vi "SMO.TimedLoop.TestLauncher.vi"() -> ()   [LabVIEW 2013, in "SMO.TimedLoop.lvclass"]
doc: "JKI State Machine Objects (SMO) 1.0.0.5\nJKI - JKI\nCopyright (c) 2016, JKI"
uses:
  SMO.TimedLoop.lvclass
  Typedefs/Data.ctl
  <vilib>/JKI/JKI SMO/SMO/Typedefs/SMOState --Enum.ctl
  <vilib>/JKI/JKI SMO/SMO/SMO.lvclass
panel:
  out "Value":T1
  in  "Setpoint":dbl(slide) scale=0.0..10.0
  out "error out":errorcluster
  in  "Stop":bool
  # "Timed Loop Test Launcher"
  # "For instructions on how to use the JKI State Machine Objects, examples and video tutorials, visit:\nhttp://jki.net/state-machine-objects/\n\nJKI State Machine Objects™\nhttp://jki.net/state-machine-objects/\nCopyright (C) 2005-2015, JKI <info@jki.net>\nALL RIGHTS RESERVED"
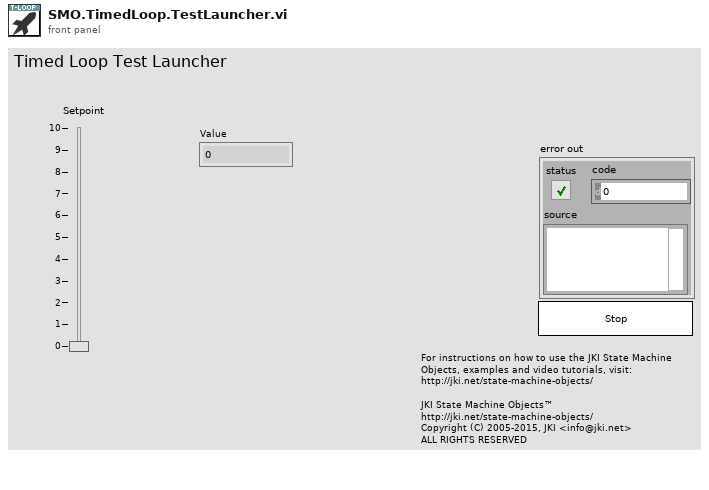
[diagram p1: front panel]
types:
  T1 = typedef "SMO.TimedLoop.lvclass/Data.ctl" = dbl
  T2 = typedef "SMO.lvclass/Public Events.ctl" = cluster{"Error":refnum<user-event>, "State":refnum<user-event>}
  T3 = typedef "SMO.TimedLoop.lvclass/PublicEvents--Cluster.ctl" = cluster{"Setpoint Changed":refnum<user-event>, "Value Changed":refnum<user-event>}
  T4 = typedef "SMO.lvclass/SMOState --Enum.ctl" = enum16{"unknown", "Created", "Started", "Stopped"}
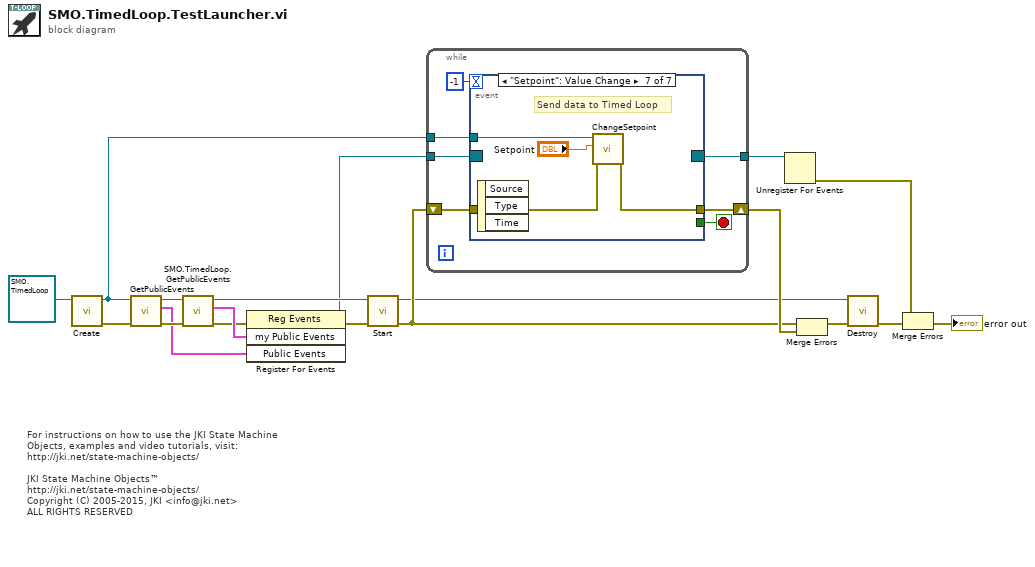
[diagram p0: block diagram]
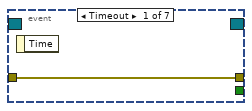
[diagram p2: hidden frame]
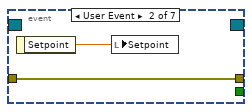
[diagram p3: hidden frame]
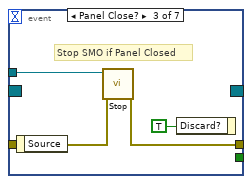
[diagram p4: hidden frame]
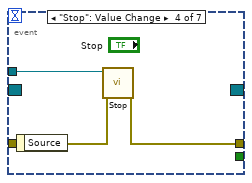
[diagram p5: hidden frame]
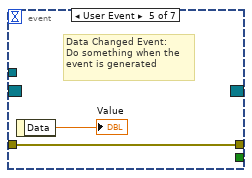
[diagram p6: hidden frame]
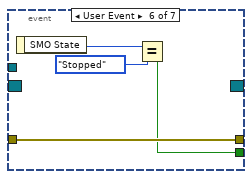
[diagram p7: hidden frame]
diagram:
  # "For instructions on how to use the JKI State Machine Objects, examples and video tutorials, visit:\nhttp://jki.net/state-machine-objects/\n\nJKI State Machine Objects™\nhttp://jki.net/state-machine-objects/\nCopyright (C) 2005-2015, JKI <info@jki.net>\nALL RIGHTS RESERVED"
  n1 = call <vilib>:"Create.vi"("SMO"=refnum<class "SMO.TimedLoop.lvclass"> refnum ("SMO.Template.lvclass")) -> ("error out"=w8:errorcluster, "SMO out"=w3:refnum<class "SMO.TimedLoop.lvclass">)  [unwired: 8 in, 1 out]
  n2 = call <vilib>:"GetPublicEvents.vi"("error in (no error)"=w8, "SMO"=w3) -> ("error out"=w7:errorcluster, "Public Events"=w2:T2, "SMO out"=w6:refnum<class "SMO.TimedLoop.lvclass">)  [unwired: 7 in]
  n3 = call "SMO.TimedLoop.GetPublicEvents.vi"("error in (no error)"=w7, "SMO.TimedLoop"=w6) -> ("error out"=w5:errorcluster, "my Public Events"=w9:T3, "SMO.TimedLoop out"=w10:refnum<class "SMO.TimedLoop.lvclass">)  [unwired: 7 in]
  n4 = register-events(error in=w5, w9, w2) -> (reference out=w1:refnum<event-registration>, error out=w4:errorcluster)  [unwired: 1 in]
  n5 = call <vilib>:"Start.vi"("error in (no error)"=w4, "SMO"=w10) -> ("error out"=w13:errorcluster, "SMO out"=w11:refnum<class "SMO.TimedLoop.lvclass">)  [unwired: 8 in]
  n6 = while {
    shift-right: [w25] -> w18
    shift-left: w13 -> [w24]
    tunnel: w1 -> [w23]
    tunnel: [w22] -> w19
    tunnel: w3 -> [w21]
    stop <- w26 stop-if-true
    n7 = event shown="[6] \"Setpoint\": Value Change" {
      selector: w23 -> [_ _ _ _ _ _ _]
      dyn-events: [_ _ _ _ _ _ _] -> w22
      timeout: -1 -> [_ _ _ _ _ _ _]
      tunnel: [_ _ _ _ _ w39 _] -> w26
      tunnel: w21 -> [_ _ w33 w36 _ _ w46]
      tunnel: [w27 w29 w32 w35 w38 w42 w43] -> w25
      tunnel: w24 -> [w27 w29 w31 w34 w38 w42 w44]
      event Timeout {
        n8 = event-data() -> ()  [unwired: 1 in, 1 out]
      }
      event User Event {
        n9 = event-data() -> ("Setpoint"=w28:T1)  [unwired: 1 in]
        n10 = local write "Setpoint"(w28) -> ()
      }
      event Panel Close? {
        # "Stop SMO if Panel Closed"
        n11 = event-data() -> ()  [unwired: 1 in, 1 out]
        n12 = call <vilib>:"Stop.vi"("error in (no error)"=w31, "SMO"=w33) -> ("error out"=w32:errorcluster)  [unwired: 8 in, 1 out]
        n13 = event-data("Discard?"=TRUE ("OK")) -> ()  [unwired: 1 in, 1 out]
      }
      event "Stop": Value Change {
        n14 = event-data() -> ()  [unwired: 1 in, 1 out]
        n15 = call <vilib>:"Stop.vi"("error in (no error)"=w34, "SMO"=w36) -> ("error out"=w35:errorcluster)  [unwired: 8 in, 1 out]
      }
      event User Event {
        # "Data Changed Event:\nDo something when the\nevent is generated"
        n16 = event-data() -> ("Data"=→"Value":T1)  [unwired: 1 in]
      }
      event User Event {
        n17 = event-data() -> ("SMO State"=w41:T4)  [unwired: 1 in]
        n18 = Equal?(x=w41, y=SMOState_--Enum."Stopped") -> (x = y?=w39:bool)
      }
      event "Setpoint": Value Change {
        # "Send data to Timed Loop"
        n19 = event-data() -> ()  [unwired: 1 in, 3 out]
        n20 = call "ChangeSetpoint.vi"("error in (no error)"=w44, "Setpoint"="Setpoint", "SMO.TimedLoop"=w46) -> ("error out"=w43:errorcluster)  [unwired: 7 in, 1 out]
      }
    }
  }
  n21 = Unregister For Events(event registration refnum=w19) -> (error out=w17:errorcluster)  [unwired: 1 in]
  n22 = Merge Errors(w13, w18) -> (w12:errorcluster)
  n23 = call <vilib>:"Destroy.vi"("error in (no error)"=w12, "SMO"=w11) -> ("error out"=w15:errorcluster)  [unwired: 9 in]
  n24 = Merge Errors(w17, w15) -> (→"error out":errorcluster)
